vi "Get Assert Name.vi"(6 "Visible Column Names":string[](array[string]), 8 "error in (no error)":errorcluster, 10 "Coords":T1, 11 "Table in":refnum<vi>) -> (0 "error out":errorcluster, 2 "Assert Name":string)   [LabVIEW 2016, in "UserInterface.lvlib" / "UserInterface.lvclass"]
uses:
  UserInterface.lvclass
  <vilib>/Utility/miscctls.llb/LVPoint32TypeDef.ctl
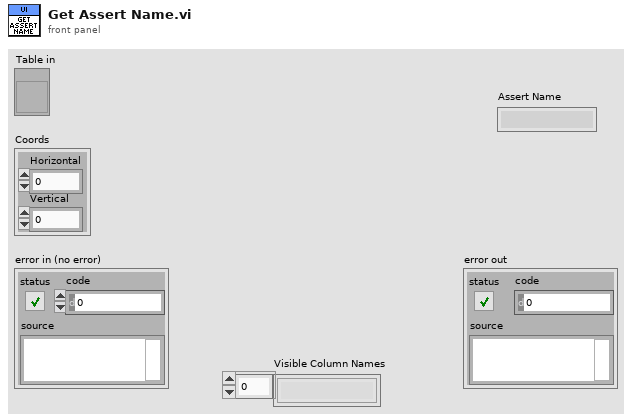
[diagram p1: front panel]
types:
  T1 = typedef "LVPoint32TypeDef.ctl" = cluster{"Horizontal":i32, "Vertical":i32}
  T2 = typedef "LVRowAndColumnTypeDef.ctl" = cluster{"Row":i32, "Column":i32}
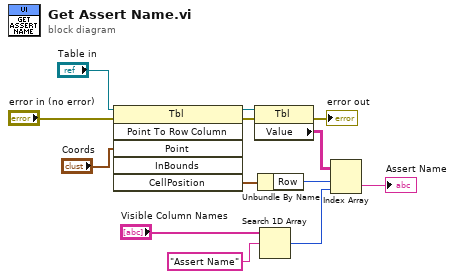
[diagram p0: block diagram]
diagram:
  n1 = invoke class="Tbl" method="Point To Row Column"(reference="Table in", error in="error in (no error)", "Point"="Coords") -> (reference out=w12:refnum<vi>, error out=w13:errorcluster, "CellPosition"=w11:T2)  [unwired: 3 in, 3 out]
  n2 = property class="Tbl"(reference=w12, error in=w13) -> (error out=→"error out":errorcluster, "Value"=w5:string[][])  [unwired: 1 out]
  n3 = Unbundle By Name(w11) -> ("Row"=w4:i32)
  n4 = Search 1D Array(1D array="Visible Column Names", element="Assert Name") -> (index of element=w3:i32)  [unwired: 1 in]
  n5 = Index Array(array=w5, index (row)=w4, index (col)=w3) -> (element=→"Assert Name":string)
